vi "RSZVB Set Sweep Segment Sweep Time.vi"(7 "Time (21.0 s)":dbl=21.0 format="%^.3e", 8 "error in (no error)":errorcluster {"code" format="%.0x"}, 9 "Segment (1)":i32=1, 10 "Channel (1)":i32=1, 11 "VISA session":refnum<visa-resource-name>) -> (0 "error out":errorcluster {"code" format="%.0x"}, 3 "dup VISA session":refnum<visa-resource-name>)   [LabVIEW 2011]
doc: "This VI sets the duration of the sweep in sweep segment no. <Segment>. At the same time, the command activates separate sweep time setting in all sweep segments.\n\nRemote-control command(s):\n[SENSe<Ch>:]SEGMent<Seg>:SWEep:TIME"
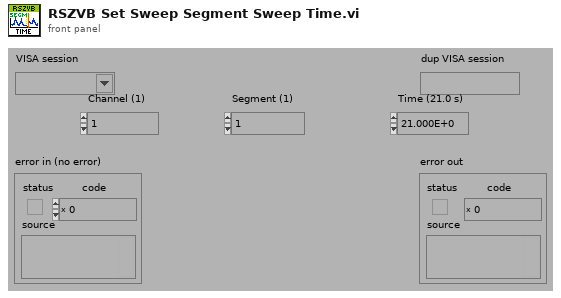
[diagram p1: front panel]
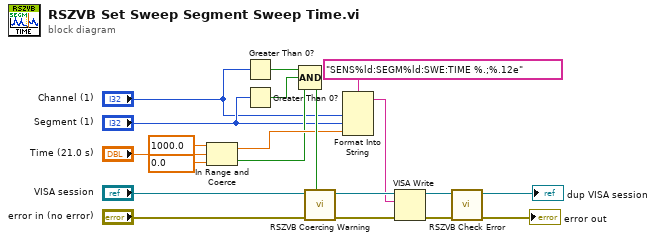
[diagram p0: block diagram]
diagram:
  n1 = In Range and Coerce(upper limit=1000.0, x="Time (21.0 s)", lower limit=0.0) -> (coerced(x)=w9:dbl, In Range?=w8:bool)
  n2 = Greater Than 0?(x="Channel (1)") -> (x > 0?=w13:bool)
  n3 = Greater Than 0?(x="Segment (1)") -> (x > 0?=w12:bool)
  n4 = Compound Arithmetic op=AND(w13, w12, w8) -> (w15:bool)
  n5 = call "RSZVB Coercing Warning.vi"("In Range?"=w15, "error in (no error)"="error in (no error)", "VISA session"="VISA session") -> ("error out"=w18:errorcluster, "dup VISA session"=w19:refnum<visa-resource-name>)  [unwired: 7 in]
  n6 = Format Into String(format string="SENS%ld:SEGM%ld:SWE:TIME %.;%.12e", "Channel (1)", "Segment (1)", w9) -> (resulting string=w14:string)  [unwired: 2 in, 1 out]
  n7 = VISA Write(VISA resource name=w19, write buffer=w14, error in (no error)=w18) -> (VISA resource name out=w16:refnum<visa-resource-name>, error out=w17:errorcluster)  [unwired: 1 out]
  n8 = call "RSZVB Check Error.vi"("error in (no error)"=w17, "VISA session"=w16) -> ("error out"=→"error out":errorcluster, "dup VISA session"=→"dup VISA session":refnum<visa-resource-name>)  [unwired: 8 in]
